vi "Write Command and Read.vi"(5 "Wait before read (0ms)":u32=5, 6 "error in (no error)":errorcluster, 7 "Bytes to read (100)":u32=100, 8 "Command":string, 9 "VISA resource name":refnum<visa-resource-name>="COM5") -> (0 "error out":errorcluster, 2 "Returned string":string, 3 "VISA resource name out":refnum<visa-resource-name>="COM5")   [LabVIEW 2020, in "Newport ESP301.lvlib"]
uses:
  Newport ESP301.lvlib
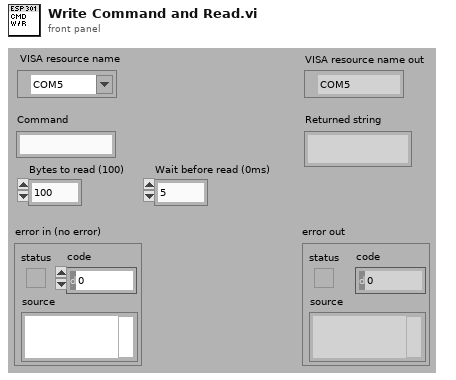
[diagram p1: front panel]
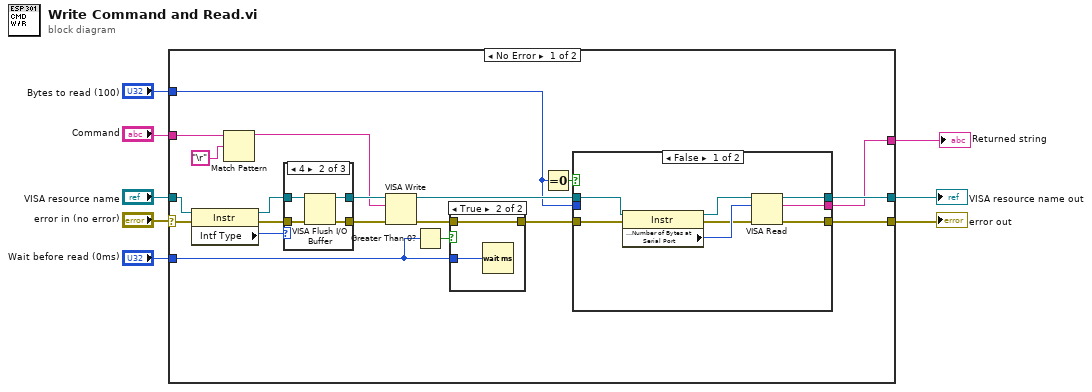
[diagram p0: block diagram]
diagram:
  n1 = case shown="No Error" "error in (no error)" {
    selector: "error in (no error)" -> [w15 w51]
    tunnel: [w28 w51] -> w7
    tunnel: "VISA resource name" -> [w17 w50]
    tunnel: [w10 w50] -> w5
    tunnel: "Command" -> [w13 _]
    tunnel: "Bytes to read (100)" -> [w20 _]
    tunnel: [w9 _] -> w2
    tunnel: "Wait before read (0ms)" -> [w22 _]
    frame No Error {
      n2 = property class="Instr"(reference=w17, error in=w15) -> (reference out=w16:refnum<visa-resource-name>, error out=w14:errorcluster, "Intf Type"=w18:u16)
      n3 = Match Pattern(string=w13, regular expression="\r") -> (before substring=w11:string)  [unwired: 4 out]
      n4 = case shown="4" w18 {
        tunnel: w16 -> [w30 w32 w36]
        tunnel: [w30 w31 w36] -> w26
        tunnel: w14 -> [w29 w34 w35]
        tunnel: [w29 w33 w35] -> w25
        frame 1 {
        }
        frame 4 {
          n5 = VISA Flush I/O Buffer(VISA resource name=w32, error in (no error)=w34) -> (VISA resource name out=w31:refnum<visa-resource-name>, error out=w33:errorcluster)  [unwired: 1 out]
        }
        frame Default {
        }
      }
      n6 = VISA Write(VISA resource name=w26, write buffer=w11, error in (no error)=w25) -> (VISA resource name out=w27:refnum<visa-resource-name>, error out=w24:errorcluster)  [unwired: 1 out]
      n7 = Greater Than 0?(x=w22) -> (x > 0?=w21:bool)
      n8 = case shown="True" w21 {
        tunnel: w24 -> [w47 w49]
        tunnel: [w47 w49] -> w23
        tunnel: w22 -> [_ w48]
        frame False {
        }
        frame True {
          n9 = Wait (ms)(milliseconds to wait=w48) -> ()  [unwired: 1 out]
        }
      }
      n10 = Equal To 0?(x=w20) -> (x = 0?=w19:bool)
      n11 = case shown="False" w19 {
        tunnel: [w44 w46] -> w28
        tunnel: w27 -> [w40 w45]
        tunnel: [w43 w45] -> w10
        tunnel: w20 -> [_ _]
        tunnel: [w42 _] -> w9
        tunnel: w23 -> [w41 w46]
        frame False {
          n12 = property class="Instr"(reference=w40, error in=w41) -> (reference out=w39:refnum<visa-resource-name>, error out=w37:errorcluster, "Serial Settings:Number of Bytes at Serial Port"=w38:u32)
          n13 = VISA Read(VISA resource name=w39, byte count=w38, error in (no error)=w37) -> (VISA resource name out=w43:refnum<visa-resource-name>, read buffer=w42:string, error out=w44:errorcluster)  [unwired: 1 out]
        }
        frame True {
        }
      }
    }
    frame Error {
    }
  }
  "error out" <- w7
  "VISA resource name out" <- w5
  "Returned string" <- w2
